vi "NumberToDeviceID-v2.vi"(9 "device raw":i32, 10 "DeviceList":T3(array[cluster]) {"Acquisition Parameters"."White level" scale=0.3..1.26 scale format="%#_2f"; "Acquisition Parameters"."Saturation" scale=0.5..1.5 scale format="%#_3f"; "Acquisition Parameters"."Contrast" scale=0.4..1.5 scale format="%#_3f"; "Acquisition Parameters"."Brightness" scale=-50.0..50.0 scale format="%#_2f"; "Correction Parameters"."Movement Type" items=["Step", "Proportionnal"]; "Target"."X Target" format="%#_5g"; "Target"."Y Target" format="%#_5g"; "Detection Parameters"."Max Intensity%" max=100 step=1}, 11 "file path in":path) -> (0 "ID":i32, 1 "CorrectConfig Cluster":T2={"Detection Parameters"={"Contrast"=0, "Treshold"=0, "Max Intensity"=0, "Max Intensity%"=0, "Rx"=0, "Ry"=0, "R%"=0.0}, "Reverse"={"Reverse X"=FALSE, "Reverse Y"=FALSE}, "Target"={"X Target"=0.0, "Y Target"=0.0}, "Region of Interest"=[-1, -1, 32000, 32000], "Correction Parameters"={"X"=5.0, "Y"=5.0, "Movement Type"=0}, "Acquisition Parameters"={"Brightness"=0.0, "Contrast"=1.0, "Saturation"=1.0, "White level"=0.7}, "Background Path"=path "", "Reference Path"=path "", "XCalibration"=[], "YCalibration"=[]} {"Acquisition Parameters"."White level" scale=0.3..1.26 scale format="%#_2f"; "Acquisition Parameters"."Saturation" scale=0.5..1.5 scale format="%#_3f"; "Acquisition Parameters"."Contrast" scale=0.4..1.5 scale format="%#_3f"; "Acquisition Parameters"."Brightness" scale=-50.0..50.0 scale format="%#_2f"; "Correction Parameters"."Movement Type" items=["Step", "Proportionnal"]; "Target"."X Target" format="%#_5g"; "Target"."Y Target" format="%#_5g"; "Detection Parameters"."Max Intensity%" max=100 step=1}, 2 "DeviceID":T1, 3 "Name":string, 4 "ImageServer":cluster{"IPAddress":string, "Port":i32})   [LabVIEW 2013]
panel:
  out "CorrectionConfig":string[](array[string])
  out "name":string
  out "Channel":i32
  out "DeviceIDOld":string[](array[string])
  # "Usefull for the scan (3.14.0 in MasterControl.vi)"
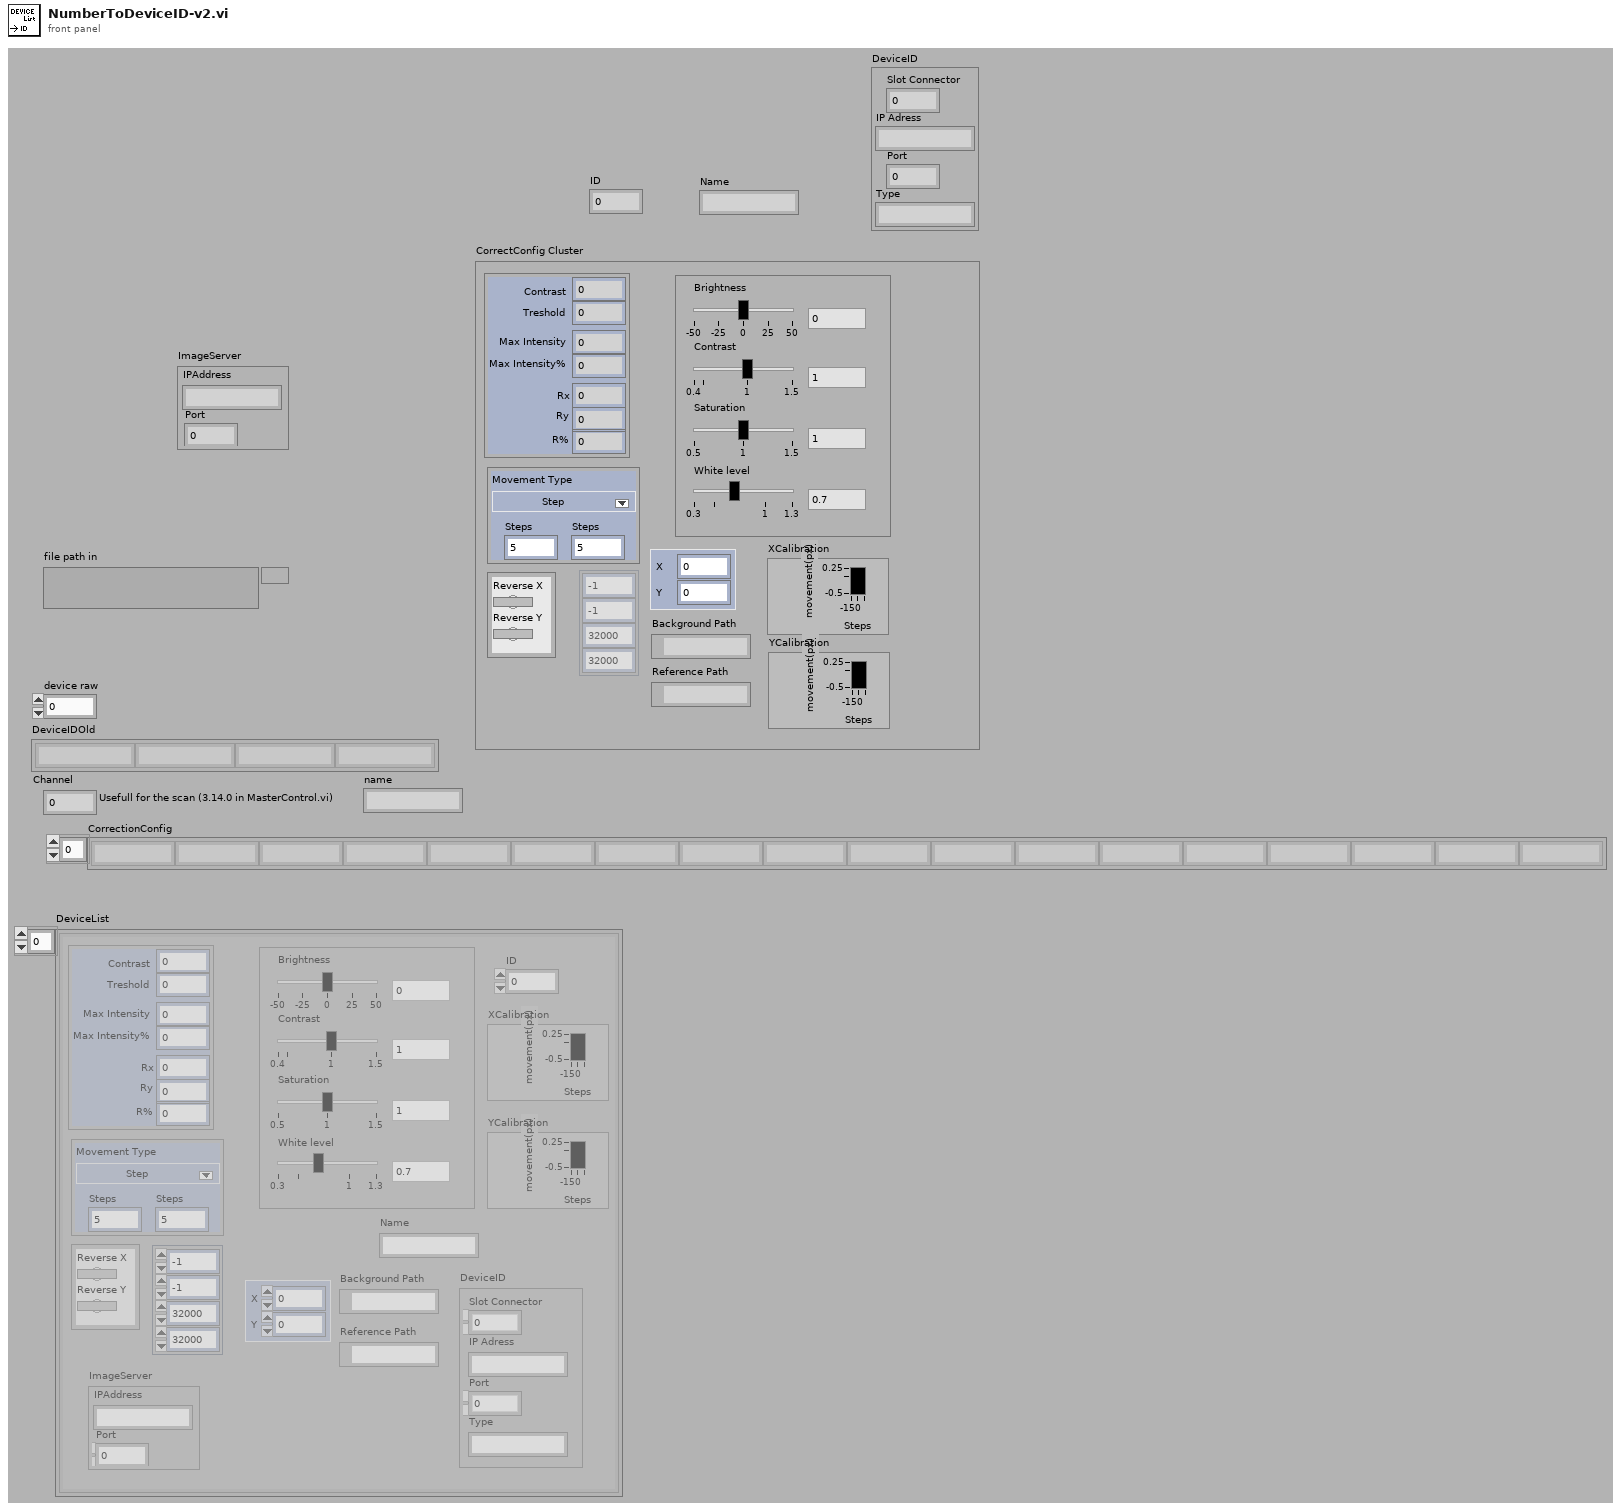
[diagram p1: front panel]
types:
  T1 = cluster{"Slot Connector":i32, "IP Adress":string, "Port":i32, "Type":string}
  T2 = cluster{"Detection Parameters":cluster{"Contrast":i32, "Treshold":u8, "Max Intensity":i32, "Max Intensity%":u8, "Rx":i32, "Ry":i32, "R%":sgl}, "Reverse":cluster{"Reverse X":bool, "Reverse Y":bool}, "Target":cluster{"X Target":sgl, "Y Target":sgl}, "Region of Interest":i32[], "Correction Parameters":cluster{"X":sgl, "Y":sgl, "Movement Type":u16}, "Acquisition Parameters":cluster{"Brightness":dbl, "Contrast":dbl, "Saturation":dbl, "White level":dbl}, "Background Path":path, "Reference Path":path, "XCalibration":cluster{dbl, dbl}[], "YCalibration":cluster{dbl, dbl}[]}
  T3 = cluster{"ID":dbl, "Name":string, "DeviceID":cluster{"Slot Connector":i32, "IP Adress":string, "Port":i32, "Type":string}, "Detection Parameters":cluster{"Contrast":i32, "Treshold":u8, "Max Intensity":i32, "Max Intensity%":u8, "Rx":i32, "Ry":i32, "R%":sgl}, "Reverse":cluster{"Reverse X":bool, "Reverse Y":bool}, "Target":cluster{"X Target":sgl, "Y Target":sgl}, "Region of Interest":i32[], "Correction Parameters":cluster{"X":sgl, "Y":sgl, "Movement Type":u16}, "Acquisition Parameters":cluster{"Brightness":dbl, "Contrast":dbl, "Saturation":dbl, "White level":dbl}, "Background Path":path, "Reference Path":path, "XCalibration":cluster{dbl, dbl}[], "YCalibration":cluster{dbl, dbl}[], "ImageServer":cluster{"IPAddress":string, "Port":i32}}[]
  T4 = cluster{"ID":dbl, "Name":string, "DeviceID":cluster{"Slot Connector":i32, "IP Adress":string, "Port":i32, "Type":string}, "Detection Parameters":cluster{"Contrast":i32, "Treshold":u8, "Max Intensity":i32, "Max Intensity%":u8, "Rx":i32, "Ry":i32, "R%":sgl}, "Reverse":cluster{"Reverse X":bool, "Reverse Y":bool}, "Target":cluster{"X Target":sgl, "Y Target":sgl}, "Region of Interest":i32[], "Correction Parameters":cluster{"X":sgl, "Y":sgl, "Movement Type":u16}, "Acquisition Parameters":cluster{"Brightness":dbl, "Contrast":dbl, "Saturation":dbl, "White level":dbl}, "Background Path":path, "Reference Path":path, "XCalibration":cluster{dbl, dbl}[], "YCalibration":cluster{dbl, dbl}[], "ImageServer":cluster{"IPAddress":string, "Port":i32}}
  T5 = cluster{"Contrast":i32, "Treshold":u8, "Max Intensity":i32, "Max Intensity%":u8, "Rx":i32, "Ry":i32, "R%":sgl}
  T6 = cluster{"Brightness":dbl, "Contrast":dbl, "Saturation":dbl, "White level":dbl}
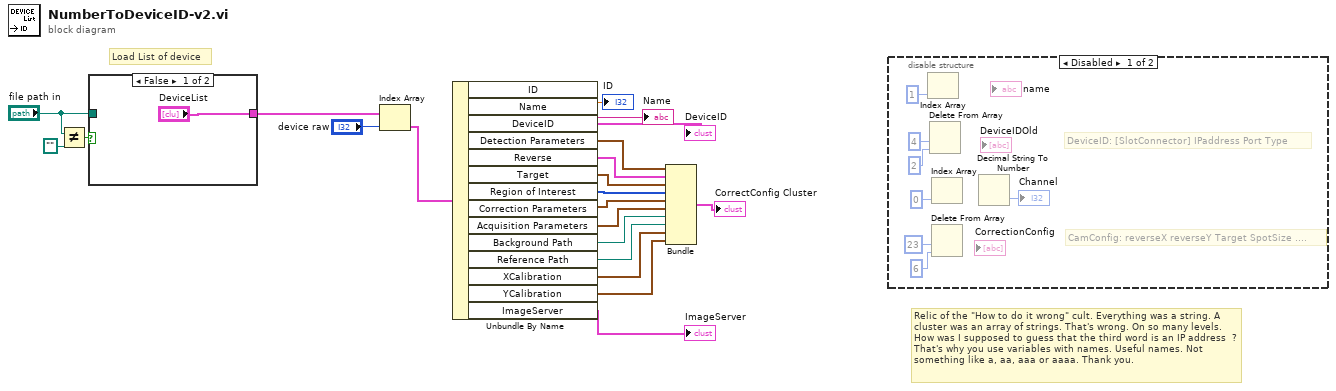
[diagram p0: block diagram]
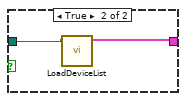
[diagram p3: hidden frame]
diagram:
  # "Relic of the \"How to do it wrong\" cult. Everything was a string. A cluster was an array of strings. That's wrong. On so many levels. How was I supposed to guess that the third word is an IP address  ? That's why you use variables with names. Useful names. Not something like a, aa, aaa or aaaa. Thank you."
  # "Load List of device"
  n1 = Not Equal?(x="file path in", y=path "") -> (x != y?=w19:bool)
  n2 = case shown="False" w19 {
    tunnel: ["DeviceList" w23] -> w16
    tunnel: "file path in" -> [_ w24]
    frame False {
    }
    frame True {
      n3 = call "LoadDeviceList.vi"("path to XML document"=w24) -> ("DeviceList"=w23:T3)  [unwired: 8 in, 2 out]
    }
  }
  n4 = Index Array(array=w16, index="device raw") -> (element=w17:T4)
  n5 = Unbundle By Name(w17) -> ("ID"=→"ID":dbl, "Name"=→"Name":string, "DeviceID"=→"DeviceID":T1, "Detection Parameters"=w14:T5, "Reverse"=w13:cluster{"Reverse X":bool, "Reverse Y":bool}, "Target"=w12:cluster{"X Target":sgl, "Y Target":sgl}, "Region of Interest"=w11:i32[], "Correction Parameters"=w10:cluster{"X":sgl, "Y":sgl, "Movement Type":u16}, "Acquisition Parameters"=w9:T6, "Background Path"=w8:path, "Reference Path"=w7:path, "XCalibration"=w3:cluster{dbl, dbl}[], "YCalibration"=w2:cluster{dbl, dbl}[], "ImageServer"=→"ImageServer":cluster{"IPAddress":string, "Port":i32})
  n6 = Bundle("Detection Parameters"=w14, "Reverse"=w13, "Target"=w12, "Region of Interest"=w11, "Correction Parameters"=w10, "Acquisition Parameters"=w9, "Background Path"=w8, "Reference Path"=w7, "XCalibration"=w3, "YCalibration"=w2) -> (→"CorrectConfig Cluster":T2)  [unwired: 1 in]
  n7 = disable-structure shown="Disabled" {
    frame Disabled {
      # "CamConfig: reverseX reverseY Target SpotSize ...."
      # "DeviceID: [SlotConnector] IPaddress Port Type"
      n8 = Index Array(index=1) -> ()  [unwired: 1 in, 1 out]
      n9 = Delete From Array(length=4, index=2 ("length")) -> ()  [unwired: 1 in, 2 out]
      n10 = Index Array(index=0) -> ()  [unwired: 1 in, 1 out]
      n11 = Delete From Array(length=23, index=6 ("length")) -> ()  [unwired: 1 in, 2 out]
      n12 = Decimal String To Number() -> (number=→"Channel":i32)  [unwired: 1 in, 3 out]
    }
    frame Enabled {
    }
  }
